vi "数据主动和反控发送2.vi"() -> ()   [LabVIEW 2016, in "数据传输系统-06.lvlib"]
uses:
  <vilib>/ptbypt/NI_PtbyPt.lvlib
panel:
  in  "N个五分钟":u32
  out "QN":string
  out "元素":cluster{"命令编码CN":string, "QN":string}[](array[cluster])
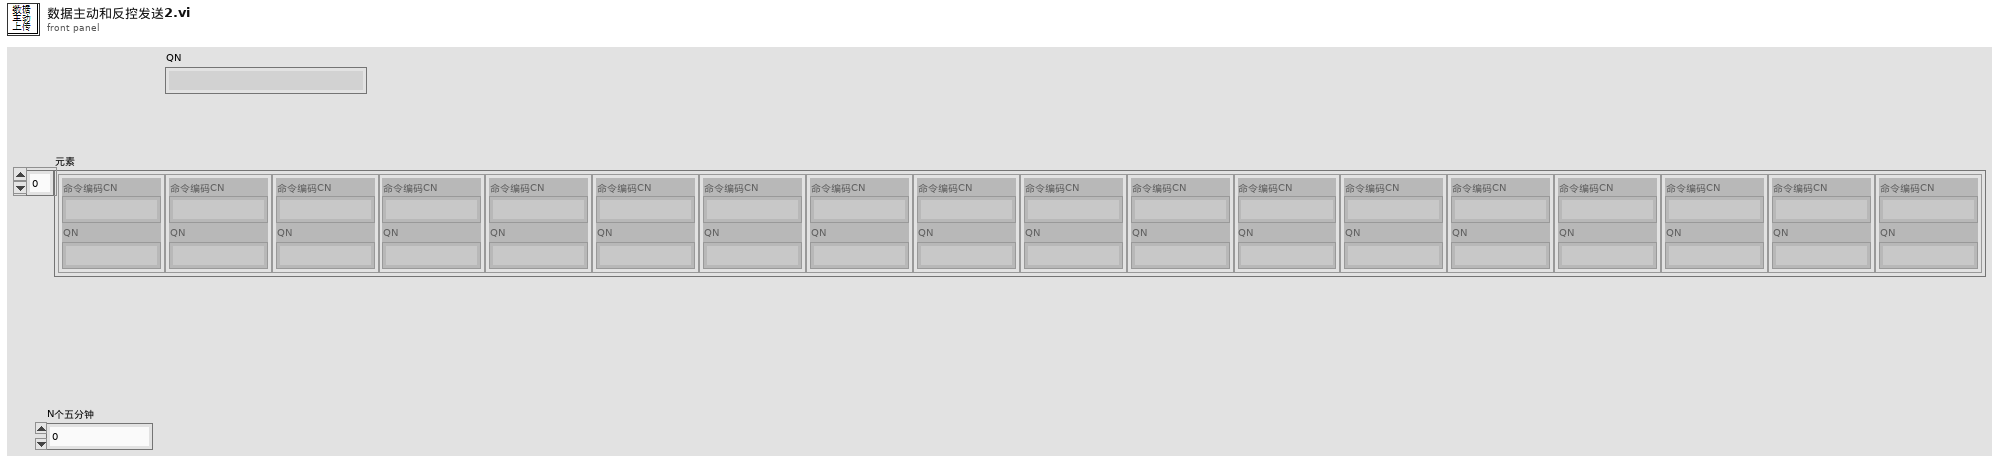
[diagram p1: front panel]
types:
  T1 = cluster{"setini":string, "sysini":string, "hechaini":string, "actualwrite":string, "actualread":string, "datasent":string, "反控命令信息队列":string, "反控与仪器交互":string}
  T2 = typedef "LVDateTimeRec.ctl" = cluster{"秒数的小数部分":dbl, "秒":i32, "分":i32, "时":i32, "日":i32, "月":i32, "年":i32, "天数（周）":i32, "天数（年）":i32, "DST":i32}
  T3 = typedef "数据传输系统-06.lvlib/应用环境.ctl" = enum16{"STD", "GB212", "婉仪平台"}
  T4 = enum16{"关闭", "星期日", "星期一", "星期二", "星期三", "星期四", "星期五", "星期六"}
  T5 = enum16{"00点", "01点", "02点", "03点", "04点", "05点", "06点", "07点", "08点", "09点", "10点", "11点", "12点", "13点", "14点", "15点", "16点", "17点", "18点", "19点", "20点", "21点", "22点", "23点"}
  T6 = cluster{"[0]":string, "[1]":string, "[2]":string, "[3]":string, "[4]":string, "[5]":string, "[6]":string, "[7]":string, "[8]":string, "[9]":string, "[10]":string, "[11]":string, "[12]":string, "[13]":string, "[14]":string, "[15]":string, "[16]":string, "[17]":string, "[18]":string, "[19]":string, "[20]":string, "[21]":string, "[22]":string, "[23]":string, "[24]":string, "[25]":string, "[26]":string, "[27]":string, "[28]":string, "[29]":string, "[30]":string, "[31]":string, "[32]":string, "[33]":string, "[34]":string, "[35]":string, "[36]":string, "[37]":string, "[38]":string, "[39]":string, "[40]":string, "[41]":string, "[42]":string, "[43]":string, "[44]":string, "[45]":string, "[46]":string, "[47]":string, "[48]":string, "[49]":string, "[50]":string, "[51]":string, "[52]":string, "[53]":string, "[54]":string, "[55]":string, "[56]":string, "[57]":string, "[58]":string, "[59]":string, "[60]":string, "[61]":string, "[62]":string, "[63]":string, "[64]":string, "[65]":string, "[66]":string, "[67]":string, "[68]":string, "[69]":string, "[70]":string, "[71]":string, "[72]":string, "[73]":string, "[74]":string, "[75]":string}
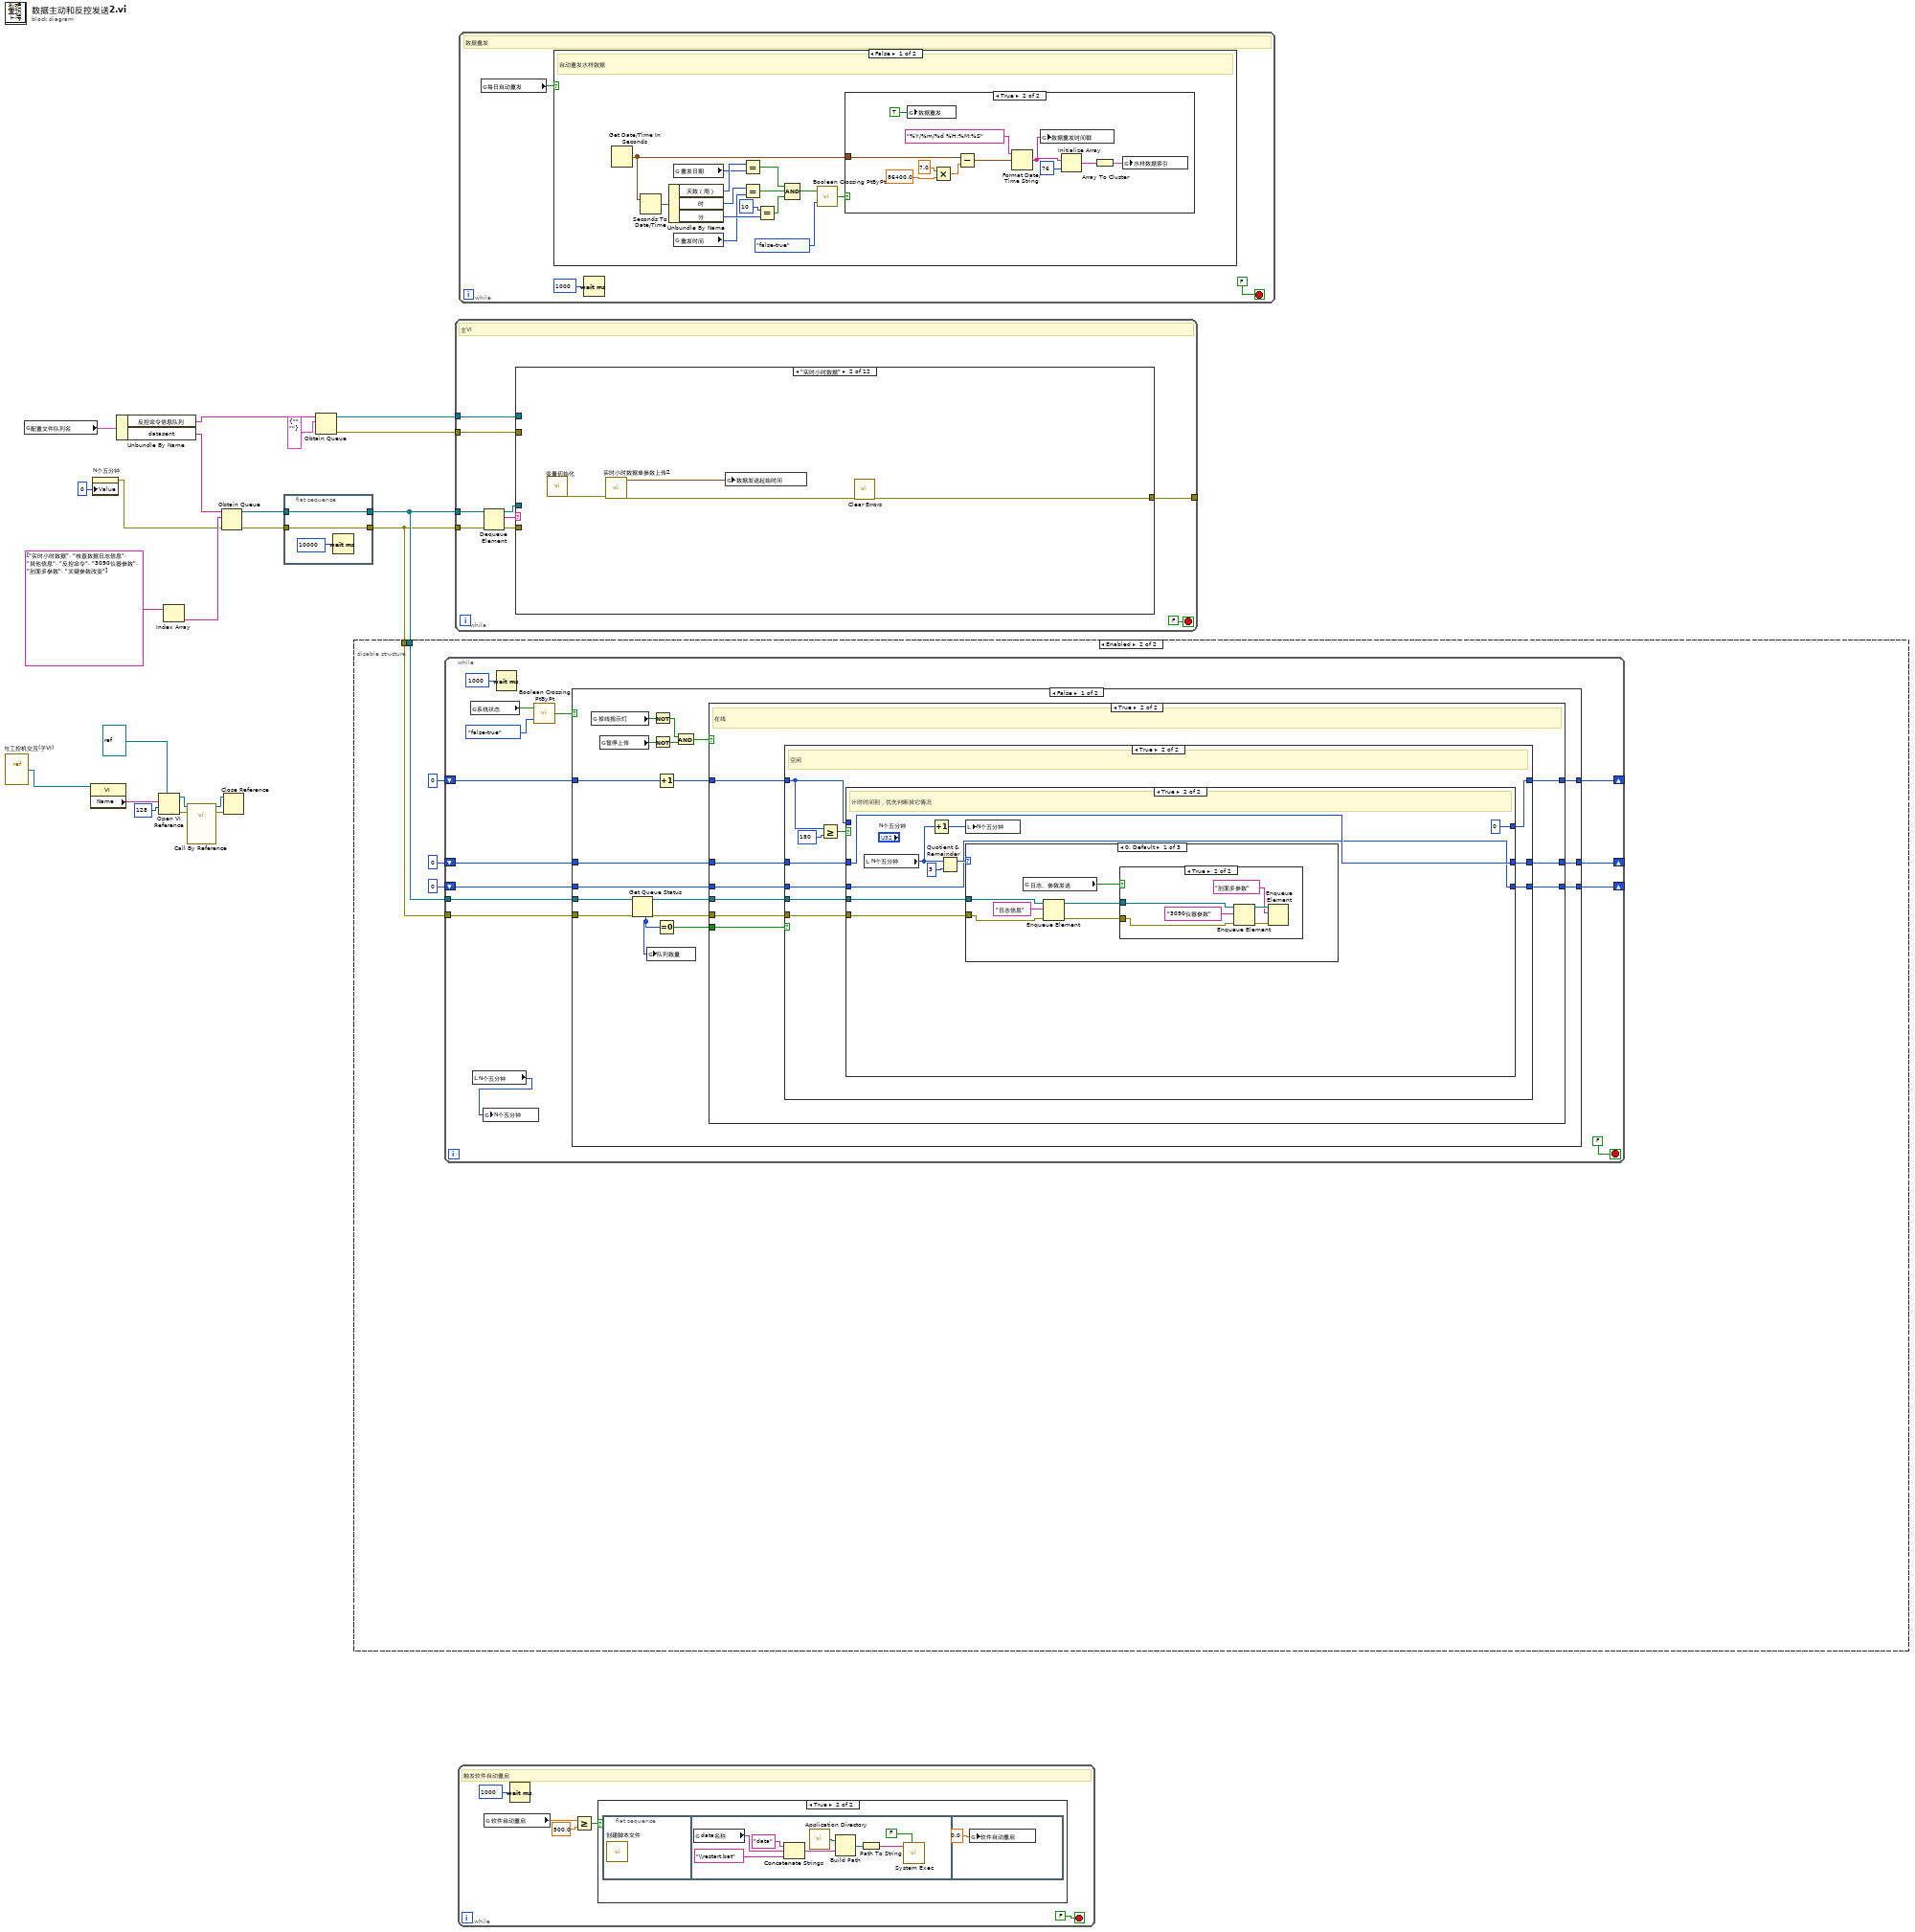
[diagram p0: block diagram]
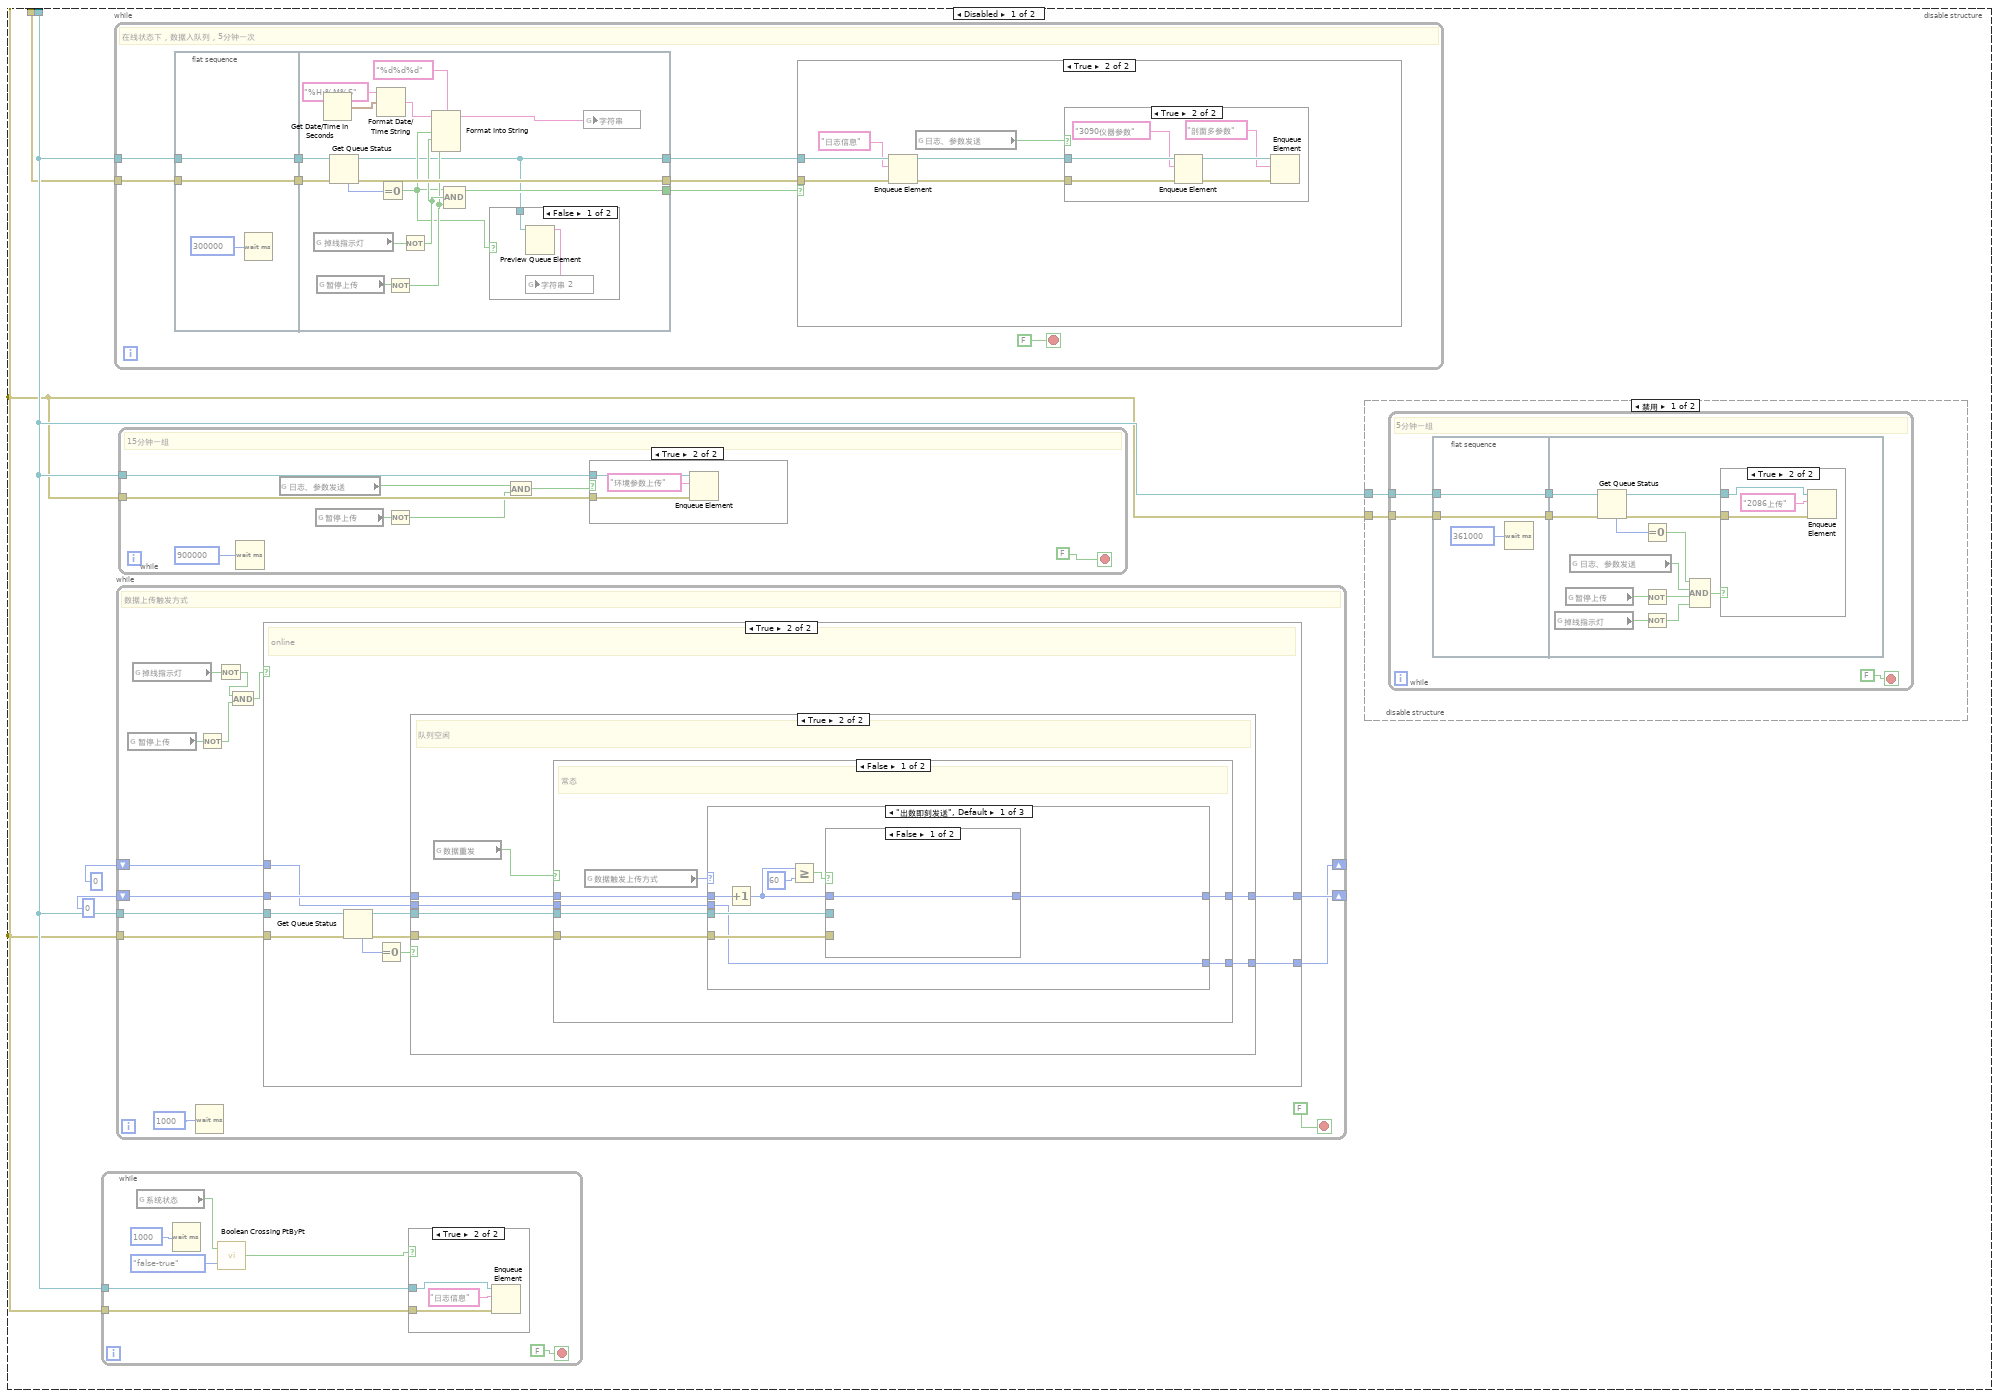
[diagram p2: hidden frame]
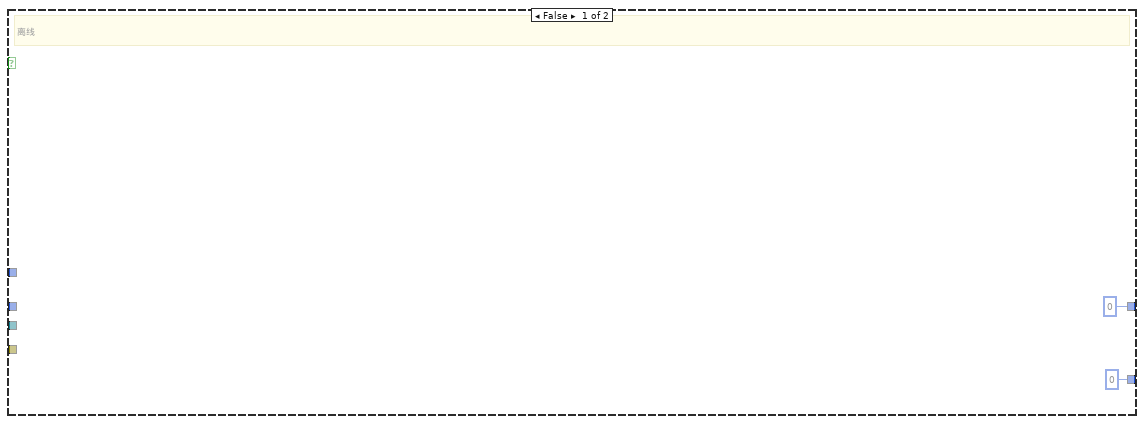
[diagram p6: hidden frame]
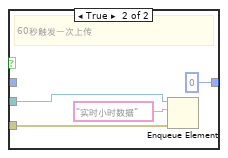
[diagram p8: hidden frame]
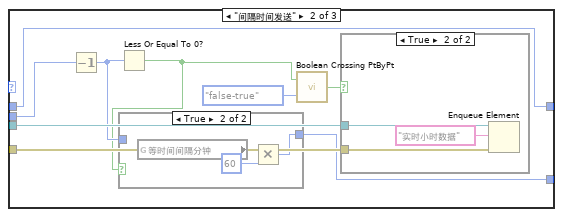
[diagram p9: hidden frame]
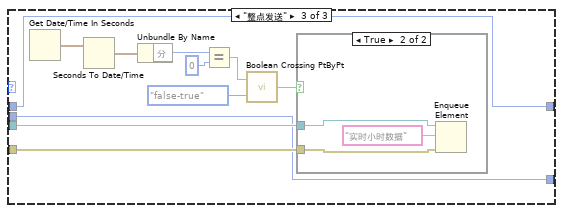
[diagram p12: hidden frame]
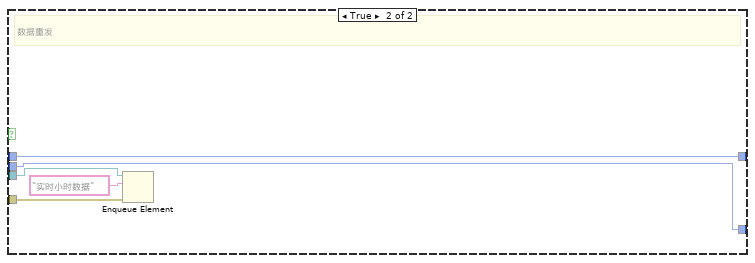
[diagram p14: hidden frame]
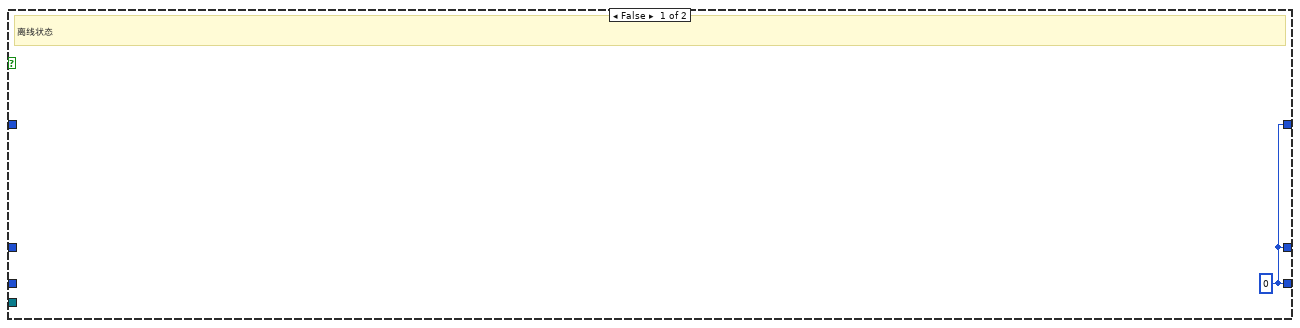
[diagram p19: hidden frame]
diagram:
  n1 = vi-ref "与工控机交互(子VI).vi"() -> (w15:refnum<vi>)
  n2 = global read "全局1.vi" "配置文件队列名"() -> (w5:T1)
  n3 = property class="VI"(reference=w15) -> ("Name"=w14:string)  [unwired: 1 in, 2 out]
  n4 = property on="N个五分钟" class="DigNum (strict)"("Value"=u32 0 ("N个五分钟")) -> (error out=w1:errorcluster)  [unwired: 2 in, 1 out]
  n5 = Unbundle By Name(w5) -> ("反控命令信息队列"=w9:string, "datasent"=w8:string)
  n6 = Open VI Reference(type specifier VI Refnum (for type only)=refnum<vi> refnum, vi path=w14, options=128 ("选项")) -> (vi reference=w12:refnum<vi>, error out=w6:errorcluster)  [unwired: 3 in]
  n7 = Index Array(array=string[] ["实时小时数据", "核查数据日志信息", "其他信息", "反控命令", "3090仪器参数", "剖面多参数", "关键参数改变"]) -> (element=w16:string)  [unwired: 1 in]
  n8 = call-by-ref "?"(reference=w12, error in=w6) -> (reference out=w10:refnum<vi>, error out=w7:errorcluster)  [unwired: 12 in]
  n9 = Obtain Queue(name (unnamed)=w8, element data type=w16, error in (no error)=w1) -> (queue out=w22:refnum<queue>, error out=w21:errorcluster)  [unwired: 2 in, 1 out]
  n10 = Close Reference(reference=w10, error in (no error)=w7) -> ()  [unwired: 1 out]
  n11 = flat-sequence {
    tunnel: w22 -> [w24]
    tunnel: [w24] -> w4
    tunnel: w21 -> [w23]
    tunnel: [w23] -> w3
    frame #0 {
      n12 = Wait (ms)(milliseconds to wait=u32 10000 ("等待时间（毫秒）")) -> ()  [unwired: 1 out]
    }
  }
  n13 = Obtain Queue(name (unnamed)=w9, element data type=cluster{"命令编码CN":string, "QN":string} {"命令编码CN"="", "QN"=""}) -> (queue out=w19:refnum<queue>, error out=w18:errorcluster)  [unwired: 3 in, 1 out]
  n14 = disable-structure shown="Enabled" {
    disable-tunnel: w4 -> [w27 w210]
    disable-tunnel: w3 -> [w26 w209]
    frame Disabled {
      n15 = while {
        tunnel: w27 -> [w57]
        tunnel: w26 -> [w56]
        stop <- FALSE stop-if-true
        n16 = global read "全局1.vi" "系统状态"() -> (w59:bool)
        n17 = Wait (ms)(milliseconds to wait=u32 1000 ("等待时间（毫秒）")) -> ()  [unwired: 1 out]
        n18 = call <vilib>:"Boolean Crossing PtByPt.vi"("direction"=enum16{"either", "false-true", "true-false"}."false-true", "input"=w59) -> ("crossing"=w55:bool)  [unwired: 1 in]
        n19 = case shown="True" w55 {
          tunnel: w57 -> [_ w62]
          tunnel: w56 -> [_ w63]
          frame False {
          }
          frame True {
            n20 = Enqueue Element(queue=w62, element="日志信息" ("元素"), error in (no error)=w63) -> ()  [unwired: 1 in, 3 out]
          }
        }
      }
      n21 = while {
        tunnel: w27 -> [w172]
        tunnel: w26 -> [w171]
        stop <- FALSE stop-if-true
        # "在线状态下，数据入队列，5分钟一次"
        n22 = flat-sequence {
          tunnel: w171 -> [w174]
          tunnel: w172 -> [w175]
          tunnel: [w175] -> w166
          tunnel: [w174] -> w165
          tunnel: [w177] -> w170
          tunnel: [w189] -> w169
          tunnel: [w187] -> w167
          tunnel: w166 -> [w191]
          tunnel: w165 -> [w190]
          frame #0 {
            n23 = Wait (ms)(milliseconds to wait=u32 300000 ("等待时间（毫秒）")) -> ()  [unwired: 1 out]
          }
          frame #1 {
            n24 = global read "全局 数据发送重叠.vi" "掉线指示灯"() -> (w188:bool)
            n25 = global read "断电保存全局.vi" "暂停上传"() -> (w186:bool)
            n26 = Get Date/Time In Seconds() -> (seconds since 1Jan1904=w184:timestamp)
            n27 = Get Queue Status(queue=w191, error in (no error)=w190) -> (queue out=w177:refnum<queue>, error out=w189:errorcluster, # elements in queue=w185:i32)  [unwired: 1 in, 5 out]
            n28 = Format Date/Time String(time format string (%c)="%H:%M%S" ("时间格式字符串(%c)"), seconds (now)=w184) -> (date/time string=w182:string)  [unwired: 1 in]
            n29 = Equal To 0?(x=w185) -> (x = 0?=w178:bool)
            n30 = Not(x=w186) -> (.not. x?=w179:bool)
            n31 = Not(x=w188) -> (.not. x?=w180:bool)
            n32 = Format Into String(format string="%d%d%d" ("格式字符串"), initial string=w182, w178, w180, w179) -> (resulting string=w176:string)  [unwired: 1 in, 1 out]
            n33 = Compound Arithmetic op=AND ("复合运算")(w178, w180, w179) -> (w187:bool)
            n34 = case shown="False" w178 {
              tunnel: w177 -> [w193 _]
              frame False {
                n35 = Preview Queue Element(queue=w193) -> (element=w192:string)  [unwired: 2 in, 3 out]
                n36 = global write "全局 水样时间.vi" "字符串 2"(w192) -> ()
              }
              frame True {
              }
            }
            n37 = global write "全局 水样时间.vi" "字符串"(w176) -> ()
          }
        }
        n38 = case shown="True" w167 {
          tunnel: w170 -> [_ w199]
          tunnel: w169 -> [_ w198]
          frame False {
          }
          frame True {
            n39 = Enqueue Element(queue=w199, element="日志信息" ("元素"), error in (no error)=w198) -> (queue out=w196:refnum<queue>, error out=w195:errorcluster)  [unwired: 1 in, 1 out]
            n40 = global read "断电保存全局.vi" "日志、参数发送"() -> (w194:bool)
            n41 = case shown="True" w194 {
              tunnel: w196 -> [_ w205]
              tunnel: w195 -> [_ w204]
              frame False {
              }
              frame True {
                n42 = Enqueue Element(queue=w205, element="3090仪器参数" ("元素"), error in (no error)=w204) -> (queue out=w202:refnum<queue>, error out=w201:errorcluster)  [unwired: 1 in, 1 out]
                n43 = Enqueue Element(queue=w202, element="剖面多参数" ("元素"), error in (no error)=w201) -> ()  [unwired: 1 in, 3 out]
              }
            }
          }
        }
      }
      n44 = while {
        tunnel: w27 -> [w72]
        tunnel: w26 -> [w71]
        shift-right: [w74] -> _
        shift-left: 0 -> [w75]
        shift-right: [w65] -> _
        shift-left: 0 -> [w66]
        stop <- FALSE stop-if-true
        # "数据上传触发方式"
        n45 = global read "断电保存全局.vi" "暂停上传"() -> (w69:bool)
        n46 = global read "全局 数据发送重叠.vi" "掉线指示灯"() -> (w76:bool)
        n47 = Wait (ms)(milliseconds to wait=u32 1000 ("等待时间（毫秒）")) -> ()  [unwired: 1 out]
        n48 = Not(x=w69) -> (.not. x?=w68:bool)
        n49 = Not(x=w76) -> (.not. x?=w70:bool)
        n50 = And(x=w70, y=w68) -> (x .and. y?=w67:bool)
        n51 = case shown="True" w67 {
          tunnel: w75 -> [_ w89]
          tunnel: [0 w88] -> w74
          tunnel: w72 -> [_ w86]
          tunnel: w71 -> [_ w85]
          tunnel: w66 -> [_ w81]
          tunnel: [0 w80] -> w65
          frame False {
            # "离线"
          }
          frame True {
            # "online"
            n52 = Get Queue Status(queue=w86, error in (no error)=w85) -> (queue out=w83:refnum<queue>, error out=w82:errorcluster, # elements in queue=w87:i32)  [unwired: 1 in, 5 out]
            n53 = Equal To 0?(x=w87) -> (x = 0?=w84:bool)
            n54 = case shown="True" w84 {
              tunnel: w83 -> [_ w98]
              tunnel: w82 -> [_ w97]
              tunnel: w89 -> [w91 w96]
              tunnel: [w91 w95] -> w88
              tunnel: w81 -> [w90 w94]
              tunnel: [w90 w93] -> w80
              frame False {
                # "队列忙碌中"
              }
              frame True {
                # "队列空闲"
                n55 = global read "断电保存全局.vi" "数据重发"() -> (w92:bool)
                n56 = case shown="False" w92 {
                  tunnel: w98 -> [w105 w152]
                  tunnel: w97 -> [w104 w151]
                  tunnel: w96 -> [w102 w150]
                  tunnel: [w101 w150] -> w95
                  tunnel: w94 -> [w100 w149]
                  tunnel: [w99 w149] -> w93
                  frame False {
                    # "常态"
                    n57 = global read "断电保存全局.vi" "数据触发上传方式"() -> (w103:enum16{"出数即刻发送", "间隔时间发送", "整点发送"})
                    n58 = case shown="\"出数即刻发送\", Default" w103 {
                      tunnel: w105 -> [w108 w126 w139]
                      tunnel: w104 -> [w107 w125 w138]
                      tunnel: w102 -> [w113 w127 w137]
                      tunnel: [w109 w127 w137] -> w101
                      tunnel: w100 -> [w106 w122 w135]
                      tunnel: [w106 w121 w135] -> w99
                      frame "出数即刻发送", Default {
                        n59 = Increment(x=w113) -> (x+1=w110:i32)
                        n60 = Greater Or Equal?(x=w110, y=60) -> (x >= y?=w111:bool)
                        n61 = case shown="False" w111 {
                          tunnel: w110 -> [w114 _]
                          tunnel: [w114 0] -> w109
                          tunnel: w108 -> [_ w116]
                          tunnel: w107 -> [_ w115]
                          frame False {
                          }
                          frame True {
                            # "60秒触发一次上传"
                            n62 = Enqueue Element(queue=w116, element="实时小时数据" ("元素"), error in (no error)=w115) -> ()  [unwired: 1 in, 3 out]
                          }
                        }
                      }
                      frame "间隔时间发送" {
                        n63 = Decrement(x=w122) -> (x-1=w120:i32)
                        n64 = Less Or Equal To 0?(x=w120) -> (x <= 0?=w119:bool)
                        n65 = case shown="True" w119 {
                          tunnel: w120 -> [w128 _]
                          tunnel: [w128 w129] -> w121
                          frame False {
                          }
                          frame True {
                            n66 = global read "断电保存全局.vi" "等时间间隔分钟"() -> (w130:i32)
                            n67 = Multiply(x=w130, y=60) -> (x*y=w129:i32)
                          }
                        }
                        n68 = call <vilib>:"Boolean Crossing PtByPt.vi"("direction"=enum16{"either", "false-true", "true-false"}."false-true", "input"=w119) -> ("crossing"=w123:bool)  [unwired: 1 in]
                        n69 = case shown="True" w123 {
                          tunnel: w126 -> [_ w133]
                          tunnel: w125 -> [_ w132]
                          frame False {
                          }
                          frame True {
                            n70 = Enqueue Element(queue=w133, element="实时小时数据" ("元素"), error in (no error)=w132) -> ()  [unwired: 1 in, 3 out]
                          }
                        }
                      }
                      frame "整点发送" {
                        n71 = Get Date/Time In Seconds() -> (seconds since 1Jan1904=w144:timestamp)
                        n72 = Seconds To Date/Time(time stamp (now)=w144) -> (date time rec=w145:T2)  [unwired: 1 in]
                        n73 = Unbundle By Name(w145) -> ("分"=w143:i32)
                        n74 = Equal?(x=w143, y=0) -> (x = y?=w141:bool)
                        n75 = call <vilib>:"Boolean Crossing PtByPt.vi"("direction"=enum16{"either", "false-true", "true-false"}."false-true", "input"=w141) -> ("crossing"=w136:bool)  [unwired: 1 in]
                        n76 = case shown="True" w136 {
                          tunnel: w139 -> [_ w147]
                          tunnel: w138 -> [_ w146]
                          frame False {
                          }
                          frame True {
                            n77 = Enqueue Element(queue=w147, element="实时小时数据" ("元素"), error in (no error)=w146) -> ()  [unwired: 1 in, 3 out]
                          }
                        }
                      }
                    }
                  }
                  frame True {
                    # "数据重发"
                    n78 = Enqueue Element(queue=w152, element="实时小时数据" ("元素"), error in (no error)=w151) -> ()  [unwired: 1 in, 3 out]
                  }
                }
              }
            }
          }
        }
      }
      n79 = while {
        tunnel: w27 -> [w159]
        tunnel: w26 -> [w158]
        stop <- FALSE stop-if-true
        # "15分钟一组"
        n80 = Wait (ms)(milliseconds to wait=u32 900000 ("等待时间（毫秒）")) -> ()  [unwired: 1 out]
        n81 = global read "断电保存全局.vi" "日志、参数发送"() -> (w156:bool)
        n82 = global read "断电保存全局.vi" "暂停上传"() -> (w157:bool)
        n83 = Not(x=w157) -> (.not. x?=w155:bool)
        n84 = And(x=w156, y=w155) -> (x .and. y?=w154:bool)
        n85 = case shown="True" w154 {
          tunnel: w159 -> [_ w163]
          tunnel: w158 -> [_ w162]
          frame False {
          }
          frame True {
            n86 = Enqueue Element(queue=w163, element="环境参数上传" ("元素"), error in (no error)=w162) -> ()  [unwired: 1 in, 3 out]
          }
        }
      }
      n87 = disable-structure shown="禁用" {
        disable-tunnel: w27 -> [w31 _]
        disable-tunnel: w26 -> [w30 _]
        frame Disabled {
          n88 = while {
            tunnel: w31 -> [w35]
            tunnel: w30 -> [w34]
            stop <- FALSE stop-if-true
            # "5分钟一组"
            n89 = flat-sequence {
              tunnel: w34 -> [w38]
              tunnel: w35 -> [w39]
              tunnel: [w39] -> w33
              tunnel: [w38] -> w32
              tunnel: w33 -> [w46]
              tunnel: w32 -> [w45]
              frame #0 {
                n90 = Wait (ms)(milliseconds to wait=u32 361000 ("等待时间（毫秒）")) -> ()  [unwired: 1 out]
              }
              frame #1 {
                n91 = global read "全局 数据发送重叠.vi" "掉线指示灯"() -> (w43:bool)
                n92 = global read "断电保存全局.vi" "暂停上传"() -> (w51:bool)
                n93 = global read "断电保存全局.vi" "日志、参数发送"() -> (w50:bool)
                n94 = Get Queue Status(queue=w46, error in (no error)=w45) -> (queue out=w44:refnum<queue>, error out=w40:errorcluster, # elements in queue=w47:i32)  [unwired: 1 in, 5 out]
                n95 = Equal To 0?(x=w47) -> (x = 0?=w41:bool)
                n96 = Not(x=w51) -> (.not. x?=w49:bool)
                n97 = Not(x=w43) -> (.not. x?=w42:bool)
                n98 = Compound Arithmetic op=AND ("复合运算")(w41, w50, w49, w42) -> (w48:bool)
                n99 = case shown="True" w48 {
                  tunnel: w44 -> [_ w53]
                  tunnel: w40 -> [_ w52]
                  frame False {
                  }
                  frame True {
                    n100 = Enqueue Element(queue=w53, element="2086上传" ("元素"), error in (no error)=w52) -> ()  [unwired: 1 in, 3 out]
                  }
                }
              }
            }
          }
        }
        frame Enabled {
        }
      }
    }
    frame Enabled {
      n101 = while {
        tunnel: w210 -> [w219]
        tunnel: w209 -> [w218]
        shift-right: [w217] -> _
        shift-left: 0 -> [w211]
        shift-right: [w216] -> _
        shift-left: 0 -> [w212]
        shift-right: [w215] -> _
        shift-left: 0 -> [w213]
        stop <- FALSE stop-if-true
        n102 = global read "全局1.vi" "系统状态"() -> (w222:bool)
        n103 = local read "N个五分钟"() -> (w214:u32)
        n104 = global write "全局 水样时间.vi" "N个五分钟"(w214) -> ()
        n105 = Wait (ms)(milliseconds to wait=u32 1000 ("等待时间（毫秒）")) -> ()  [unwired: 1 out]
        n106 = call <vilib>:"Boolean Crossing PtByPt.vi"("direction"=enum16{"either", "false-true", "true-false"}."false-true", "input"=w222) -> ("crossing"=w220:bool)  [unwired: 1 in]
        n107 = case shown="False" w220 {
          tunnel: w219 -> [w230 w360]
          tunnel: w218 -> [w229 w361]
          tunnel: [w237 w359] -> w217
          tunnel: [w236 w358] -> w216
          tunnel: w211 -> [w235 w359]
          tunnel: w212 -> [w234 w358]
          tunnel: w213 -> [w233 w357]
          tunnel: [w231 w357] -> w215
          frame False {
            n108 = global read "全局 数据发送重叠.vi" "掉线指示灯"() -> (w242:bool)
            n109 = global read "断电保存全局.vi" "暂停上传"() -> (w240:bool)
            n110 = Get Queue Status(queue=w230, error in (no error)=w229) -> (queue out=w228:refnum<queue>, error out=w227:errorcluster, # elements in queue=w225:i32)  [unwired: 1 in, 5 out]
            n111 = global write "全局 水样时间.vi" "队列数量"(w225) -> ()
            n112 = Not(x=w242) -> (.not. x?=w241:bool)
            n113 = Not(x=w240) -> (.not. x?=w239:bool)
            n114 = Increment(x=w233) -> (x+1=w232:i32)
            n115 = Equal To 0?(x=w225) -> (x = 0?=w226:bool)
            n116 = And(x=w241, y=w239) -> (x .and. y?=w238:bool)
            n117 = case shown="True" w238 {
              tunnel: [w243 w251] -> w237
              tunnel: [w243 w249] -> w236
              tunnel: w228 -> [_ w246]
              tunnel: w235 -> [_ w252]
              tunnel: w234 -> [_ w250]
              tunnel: w232 -> [_ w248]
              tunnel: [w243 w247] -> w231
              tunnel: w227 -> [_ w245]
              tunnel: w226 -> [_ w244]
              frame False {
                w243 = 0
                # "离线状态"
              }
              frame True {
                # "在线"
                n118 = case shown="True" w244 {
                  tunnel: w252 -> [w255 w261]
                  tunnel: [w255 w260] -> w251
                  tunnel: w250 -> [w254 w263]
                  tunnel: [w254 w262] -> w249
                  tunnel: w246 -> [_ w265]
                  tunnel: w245 -> [_ w264]
                  tunnel: w248 -> [w253 w256]
                  tunnel: [w253 w257] -> w247
                  frame False {
                    # "忙碌"
                  }
                  frame True {
                    # "空闲"
                    n119 = Greater Or Equal?(x=w256, y=180) -> (x >= y?=w258:bool)
                    n120 = case shown="True" w258 {
                      tunnel: w265 -> [w272 w331]
                      tunnel: w264 -> [w271 w330]
                      tunnel: w263 -> [w270 w337]
                      tunnel: [w269 w337] -> w262
                      tunnel: w261 -> [w268 w329]
                      tunnel: [w267 w329] -> w260
                      tunnel: [w266 0] -> w257
                      tunnel: w256 -> [w266 _]
                      frame False {
                        # "五分钟计时未到"
                        n121 = global read "断电保存全局.vi" "数据重发"() -> (w273:bool)
                        n122 = case shown="False" w273 {
                          tunnel: w272 -> [w278 w328]
                          tunnel: w271 -> [w277 w327]
                          tunnel: w270 -> [w279 w324]
                          tunnel: [w276 w324] -> w269
                          tunnel: w268 -> [w275 w325]
                          tunnel: [w274 w325] -> w267
                          frame False {
                            n123 = global read "断电保存全局.vi" "数据触发上传方式"() -> (w280:enum16{"出数即刻发送", "间隔时间发送", "整点发送"})
                            n124 = case shown="\"出数即刻发送\", Default" w280 {
                              tunnel: w279 -> [w288 w294 w310]
                              tunnel: w278 -> [w285 w297 w313]
                              tunnel: w277 -> [w284 w296 w312]
                              tunnel: [w283 w294 w310] -> w276
                              tunnel: w275 -> [w282 w301 w311]
                              tunnel: [w282 w295 w311] -> w274
                              frame "出数即刻发送", Default {
                                n125 = Increment(x=w288) -> (x+1=w281:i32)
                                n126 = Greater Or Equal?(x=w281, y=60) -> (x >= y?=w286:bool)
                                n127 = case shown="True" w286 {
                                tunnel: w285 -> [_ w293]
                                tunnel: w284 -> [_ w292]
                                tunnel: [w289 0] -> w283
                                tunnel: w281 -> [w289 _]
                                frame False {
                                }
                                frame True {
                                n128 = Enqueue Element(queue=w293, element="实时小时数据", error in (no error)=w292) -> ()  [unwired: 1 in, 3 out]
                                }
                                }
                              }
                              frame "间隔时间发送" {
                                n129 = Decrement(x=w301) -> (x-1=w300:i32)
                                n130 = Less Or Equal To 0?(x=w300) -> (x <= 0?=w299:bool)
                                n131 = case shown="True" w299 {
                                tunnel: w300 -> [w306 _]
                                tunnel: [w306 w307] -> w295
                                frame False {
                                }
                                frame True {
                                n132 = global read "断电保存全局.vi" "等时间间隔分钟"() -> (w308:i32)
                                n133 = Multiply(x=w308, y=60) -> (x*y=w307:i32)
                                }
                                }
                                n134 = call <vilib>:"Boolean Crossing PtByPt.vi"("direction"=enum16{"either", "false-true", "true-false"}."false-true", "input"=w299) -> ("crossing"=w298:bool)  [unwired: 1 in]
                                n135 = case shown="True" w298 {
                                tunnel: w297 -> [_ w304]
                                tunnel: w296 -> [_ w303]
                                frame False {
                                }
                                frame True {
                                n136 = Enqueue Element(queue=w304, element="实时小时数据" ("元素"), error in (no error)=w303) -> ()  [unwired: 1 in, 3 out]
                                }
                                }
                              }
                              frame "整点发送" {
                                n137 = Get Date/Time In Seconds() -> (seconds since 1Jan1904=w316:timestamp)
                                n138 = Seconds To Date/Time(time stamp (now)=w316) -> (date time rec=w315:T2)  [unwired: 1 in]
                                n139 = Unbundle By Name(w315) -> ("分"=w317:i32)
                                n140 = Equal?(x=w317, y=0) -> (x = y?=w319:bool)
                                n141 = call <vilib>:"Boolean Crossing PtByPt.vi"("direction"=enum16{"either", "false-true", "true-false"}."false-true", "input"=w319) -> ("crossing"=w314:bool)  [unwired: 1 in]
                                n142 = case shown="True" w314 {
                                tunnel: w313 -> [_ w322]
                                tunnel: w312 -> [_ w321]
                                frame False {
                                }
                                frame True {
                                n143 = Enqueue Element(queue=w322, element="实时小时数据" ("元素"), error in (no error)=w321) -> ()  [unwired: 1 in, 3 out]
                                }
                                }
                              }
                            }
                          }
                          frame True {
                            n144 = Enqueue Element(queue=w328, element="实时小时数据" ("元素"), error in (no error)=w327) -> ()  [unwired: 1 in, 3 out]
                          }
                        }
                      }
                      frame True {
                        # "计时时间到，优先判断其它情况"
                        n145 = local read "N个五分钟"() -> (w332:u32)
                        n146 = Increment(x=w332) -> (x+1=w333:u32)
                        n147 = Quotient & Remainder(x=w332, y=u32 3) -> (x-y*floor(x/y)=w334:u32)  [unwired: 1 out]
                        n148 = local write "N个五分钟"(w333) -> ()
                        n149 = case shown="0, Default" w334 {
                          tunnel: w331 -> [w339 w352 w354]
                          tunnel: w330 -> [w338 w351 w355]
                          frame 0, Default {
                            n150 = global read "断电保存全局.vi" "日志、参数发送"() -> (w343:bool)
                            n151 = Enqueue Element(queue=w339, element="日志信息" ("元素"), error in (no error)=w338) -> (queue out=w341:refnum<queue>, error out=w342:errorcluster)  [unwired: 1 in, 1 out]
                            n152 = case shown="True" w343 {
                              tunnel: w341 -> [_ w349]
                              tunnel: w342 -> [_ w348]
                              frame False {
                              }
                              frame True {
                                n153 = Enqueue Element(queue=w349, element="3090仪器参数" ("元素"), error in (no error)=w348) -> (queue out=w346:refnum<queue>, error out=w345:errorcluster)  [unwired: 1 in, 1 out]
                                n154 = Enqueue Element(queue=w346, element="剖面多参数" ("元素"), error in (no error)=w345) -> ()  [unwired: 1 in, 3 out]
                              }
                            }
                          }
                          frame 1 {
                            n155 = Enqueue Element(queue=w352, element="2086上传" ("元素"), error in (no error)=w351) -> ()  [unwired: 1 in, 3 out]
                            n156 = global write "全局1.vi" "2086上传"(TRUE ("2086上传")) -> ()
                          }
                          frame 2 {
                            n157 = Enqueue Element(queue=w354, element="环境参数上传" ("元素"), error in (no error)=w355) -> ()  [unwired: 1 in, 3 out]
                          }
                        }
                      }
                    }
                  }
                }
              }
            }
          }
          frame True {
            n158 = Enqueue Element(queue=w360, element="日志信息" ("元素"), error in (no error)=w361) -> ()  [unwired: 1 in, 3 out]
          }
        }
      }
    }
  }
  n159 = while {
    tunnel: w4 -> [w365]
    tunnel: w3 -> [w364]
    tunnel: w19 -> [w367]
    tunnel: w18 -> [w366]
    tunnel: [w363] -> _
    stop <- FALSE stop-if-true
    # "主VI"
    n160 = Dequeue Element(queue=w365, error in (no error)=w364) -> (queue out=w369:refnum<queue>, element=w370:string, error out=w368:errorcluster)  [unwired: 1 in, 1 out]
    n161 = case shown="\"实时小时数据\"" w370 {
      tunnel: w369 -> [_ _ w378 _ _ _ _ w400 _ _ _ _]
      tunnel: w368 -> [_ _ _ _ _ _ _ w399 _ _ _ _]
      tunnel: w367 -> [_ _ _ _ _ _ _ w407 _ _ _ _]
      tunnel: w366 -> [_ _ _ _ _ _ _ w406 _ _ _ _]
      tunnel: [_ w372 w377 w384 w390 w395 _ _ w420 w426 w433 _] -> w363
      frame Default {
      }
      frame "实时小时数据" {
        n162 = call "变量初始化.vi"() -> ("错误输出"=w373:errorcluster)  [unwired: 11 in]
        n163 = call "实时小时数据单参数上传2.vi"("错误输入（无错误）"=w373) -> ("数据发送起始时间"=w375:timestamp, "error out"=w374:errorcluster)  [unwired: 13 in]
        n164 = global write "全局1.vi" "数据发送起始时间"(w375) -> ()
        n165 = call <vilib>:"Clear Errors.vi"("error in (no error)"=w374) -> ("error out"=w372:errorcluster)  [unwired: 5 in, 1 out]
      }
      frame "日志信息" {
        n166 = call "日志信息出发送队列 (子VI).vi"("queue out"=w378) -> ("错误输出"=w376:errorcluster)  [unwired: 10 in]
        n167 = call <vilib>:"Clear Errors.vi"("error in (no error)"=w376) -> ("error out"=w377:errorcluster)  [unwired: 5 in, 1 out]
      }
      frame "关键参数改变" {
        n168 = global read "断电保存全局.vi" "仪器参数发送"() -> (w382:bool)
        n169 = global read "断电保存全局.vi" "应用环境"() -> (w383:T3)
        n170 = Equal?(x=w383, y=应用环境."STD" ("应用环境")) -> (x = y?=w381:bool)
        n171 = And(x=w382, y=w381) -> (x .and. y?=w380:bool)
        n172 = case shown="True" w380 {
          tunnel: [_ w385] -> w384
          frame False {
          }
          frame True {
            n173 = call "仪器参数改变发送 (子VI).vi"() -> ("错误输出"=w386:errorcluster)  [unwired: 11 in]
            n174 = call "采配水仪器参数改变发送 (子VI).vi"("错误输入"=w386) -> ("错误输出"=w385:errorcluster)  [unwired: 10 in]
          }
        }
      }
      frame "校准信息改变" {
        n175 = global read "断电保存全局.vi" "应用环境"() -> (w389:T3)
        n176 = Equal?(x=w389, y=应用环境."STD" ("应用环境")) -> (x = y?=w388:bool)
        n177 = case shown="True" w388 {
          tunnel: [_ w391] -> w390
          frame False {
          }
          frame True {
            n178 = call "校准信息改变发送 (子VI).vi"() -> ("错误输出"=w391:errorcluster)  [unwired: 11 in]
          }
        }
      }
      frame "3201告警信息改变" {
        n179 = global read "断电保存全局.vi" "应用环境"() -> (w394:T3)
        n180 = Equal?(x=w394, y=应用环境."婉仪平台") -> (x = y?=w393:bool)
        n181 = case shown="True" w393 {
          tunnel: [_ w396] -> w395
          frame False {
          }
          frame True {
            n182 = call "3201告警信息改变发送 (子VI).vi"() -> ("错误输出"=w396:errorcluster)  [unwired: 11 in]
          }
        }
      }
      frame "其他信息" {
      }
      frame "反控命令" {
        n183 = Get Queue Status(queue=w407, return elements? (F)=TRUE ("返回元素？(F)"), error in (no error)=w406) -> (elements=→"元素":cluster{"命令编码CN":string, "QN":string}[])  [unwired: 7 out]
        n184 = Dequeue Element(queue=w407, error in (no error)=w406) -> (element=w403:cluster{"命令编码CN":string, "QN":string})  [unwired: 1 in, 3 out]
        n185 = Unbundle By Name(w403) -> ("命令编码CN"=w397:string, "QN"=w398:string)
        "QN" <- w398
        n186 = global read "全局1.vi" "数据"() -> (w405:string)
        n187 = call "读取反控数据解析(子VI).vi"("数据"=w405, "命令编码CN"=w397) -> ("反控命令错误？"=w404:bool)  [unwired: 8 in, 1 out]
        n188 = case shown="False" w404 {
          tunnel: w398 -> [w412 _]
          tunnel: w400 -> [w410 _]
          tunnel: w399 -> [w409 _]
          tunnel: w397 -> [w408 _]
          frame False {
            # "反控命令正确"
            n189 = call "反控数据上传(子VI).vi"("QN"=w412) -> ("error out"=w411:errorcluster)  [unwired: 10 in]
            n190 = case shown="No Error" w411 {
              tunnel: w410 -> [w415 _]
              tunnel: w409 -> [w414 _]
              tunnel: w408 -> [w413 _]
              frame No Error {
                n191 = case shown="\"2084\", \"3056\"" w413 {
                  tunnel: w415 -> [_ w418]
                  tunnel: w414 -> [_ w417]
                  frame "假", Default {
                  }
                  frame "2084", "3056" {
                    n192 = Enqueue Element(queue=w418, element="日志信息" ("元素"), error in (no error)=w417) -> ()  [unwired: 1 in, 3 out]
                  }
                }
              }
              frame Error {
              }
            }
          }
          frame True {
            # "反控命令错误"
          }
        }
      }
      frame "3090仪器参数" {
        n193 = global read "断电保存全局.vi" "应用环境"() -> (w419:T3)
        n194 = case shown="\"STD\"" w419 {
          tunnel: [w421 _] -> w420
          frame "STD" {
            n195 = call "3090仪器参数上传.vi"() -> ("error out"=w422:errorcluster)  [unwired: 15 in]
            n196 = call "变量初始化.vi"("错误输入（无错误）"=w422) -> ("错误输出"=w421:errorcluster)  [unwired: 10 in]
          }
          frame "GB212", Default {
          }
        }
      }
      frame "剖面多参数" {
        n197 = global read "断电保存全局.vi" "应用环境"() -> (w425:T3)
        n198 = call "剖面多参数上传.vi"() -> ("error out"=w424:errorcluster)  [unwired: 15 in]
        n199 = call <vilib>:"Clear Errors.vi"("error in (no error)"=w424) -> ("error out"=w423:errorcluster)  [unwired: 5 in, 1 out]
        n200 = case shown="\"STD\"" w425 {
          tunnel: [w428 w429 w432] -> w426
          tunnel: w423 -> [w427 w429 w431]
          frame "STD" {
            n201 = call "新剖面数据上传.vi"("错误输入（无错误）"=w427) -> ("error out"=w428:errorcluster)  [unwired: 14 in]
          }
          frame "GB212", Default {
            n202 = global write "断电保存全局.vi" "剖面数据重发"(FALSE ("剖面数据重发")) -> ()
          }
          frame "婉仪平台" {
            n203 = call "新剖面数据上传.vi"("错误输入（无错误）"=w431) -> ("error out"=w432:errorcluster)  [unwired: 14 in]
          }
        }
      }
      frame "环境参数上传" {
        n204 = call "环境参数上传.vi"() -> ("error out"=w433:errorcluster)  [unwired: 15 in]
      }
      frame "2086上传" {
        n205 = flat-sequence {
          frame #0 {
            n206 = call "2086发送2.vi"() -> ()  [unwired: 12 in]
          }
          frame #1 {
            n207 = call "2086组合发送波浪仪.vi"() -> ()  [unwired: 12 in]
          }
          frame #2 {
            n208 = global write "全局1.vi" "2086上传"(FALSE ("2086上传")) -> ()
          }
        }
      }
    }
  }
  n209 = while {
    stop <- FALSE stop-if-true
    # "触发软件自动重启"
    n210 = global read "全局1.vi" "软件自动重启"() -> (w437:dbl)
    n211 = Wait (ms)(milliseconds to wait=u32 1000 ("等待时间（毫秒）")) -> ()  [unwired: 1 out]
    n212 = Greater Or Equal?(x=w437, y=500.0) -> (x >= y?=w435:bool)
    n213 = case shown="True" w435 {
      frame False {
      }
      frame True {
        n214 = flat-sequence {
          frame #0 {
            n215 = call "创建脚本文件.vi"() -> ()  [unwired: 11 in, 1 out]
          }
          frame #1 {
            n216 = global read "断电保存全局.vi" "data名称"() -> (w442:string)
            n217 = Concatenate Strings("data" ("名称或相对路径"), w442, "\\restart.bat" ("字符串")) -> (w440:string)
            n218 = call <vilib>:"Application Directory.vi"() -> ("Application Directory"=w446:path)
            n219 = Build Path(base path=w446, name or relative path=w440) -> (appended path=w447:path)
            n220 = Path To String(path=w447) -> (string=w444:string)
            n221 = call <vilib>:"System Exec.vi"("wait until completion? (T)"=FALSE, "command line"=w444) -> ()  [unwired: 6 in, 4 out]
          }
          frame #2 {
            n222 = global write "全局1.vi" "软件自动重启"(0.0 ("软件自动重启")) -> ()
          }
        }
      }
    }
  }
  n223 = while {
    stop <- FALSE stop-if-true
    # "数据重发"
    n224 = global read "断电保存全局.vi" "每日自动重发"() -> (w450:bool)
    n225 = case shown="False" w450 {
      frame False {
        # "自动重发水样数据"
        n226 = Get Date/Time In Seconds() -> (seconds since 1Jan1904=w453:timestamp)
        n227 = Seconds To Date/Time(time stamp (now)=w453) -> (date time rec=w460:T2)  [unwired: 1 in]
        n228 = Unbundle By Name(w460) -> ("天数（周）"=w465:i32, "时"=w456:i32, "分"=w464:i32)
        n229 = global read "断电保存全局.vi" "重发日期"() -> (w455:T4)
        n230 = global read "断电保存全局.vi" "重发时间"() -> (w454:T5)
        n231 = Equal?(x=w465, y=w455) -> (x = y?=w463:bool)
        n232 = Equal?(x=w456, y=w454) -> (x = y?=w462:bool)
        n233 = Equal?(x=10, y=w464) -> (x = y?=w461:bool)
        n234 = Compound Arithmetic op=AND ("复合运算")(w463, w462, w461) -> (w459:bool)
        n235 = call <vilib>:"Boolean Crossing PtByPt.vi"("direction"=enum16{"either", "false-true", "true-false"}."false-true", "input"=w459) -> ("crossing"=w458:bool)  [unwired: 1 in]
        n236 = case shown="True" w458 {
          tunnel: w453 -> [_ w467]
          frame False {
          }
          frame True {
            n237 = global write "断电保存全局.vi" "数据重发"(TRUE ("数据重发")) -> ()
            n238 = Multiply(x=7.0, y=86400.0) -> (x*y=w469:dbl)
            n239 = Subtract(x=w467, y=w469) -> (x-y=w466:timestamp)
            n240 = Format Date/Time String(time format string (%c)="%Y/%m/%d %H:%M:%S" ("时间格式字符串(%c)"), seconds (now)=w466) -> (date/time string=w471:string)  [unwired: 1 in]
            n241 = global write "断电保存全局.vi" "数据重发时间戳"(w471) -> ()
            n242 = Initialize Array(w471, 76 ("维数大小")) -> (w473:string[])
            n243 = Array To Cluster(array=w473) -> (cluster=w472:T6)
            n244 = global write "全局 水样时间.vi" "水样数据索引"(w472) -> ()
          }
        }
      }
      frame True {
        n245 = Get Date/Time In Seconds() -> (seconds since 1Jan1904=w477:timestamp)
        n246 = Seconds To Date/Time(time stamp (now)=w477) -> (date time rec=w484:T2)  [unwired: 1 in]
        n247 = global read "断电保存全局.vi" "重发时间"() -> (w479:T5)
        n248 = Unbundle By Name(w484) -> ("时"=w480:i32, "分"=w487:i32)
        n249 = Equal?(x=w480, y=w479) -> (x = y?=w486:bool)
        n250 = Equal?(x=10, y=w487) -> (x = y?=w485:bool)
        n251 = Compound Arithmetic op=AND ("复合运算")(w486, w485) -> (w483:bool)
        n252 = call <vilib>:"Boolean Crossing PtByPt.vi"("direction"=enum16{"either", "false-true", "true-false"}."false-true", "input"=w483) -> ("crossing"=w482:bool)  [unwired: 1 in]
        n253 = case shown="True" w482 {
          tunnel: w477 -> [_ w489]
          frame False {
          }
          frame True {
            n254 = global write "断电保存全局.vi" "数据重发"(TRUE ("数据重发")) -> ()
            n255 = Subtract(x=w489, y=86400.0) -> (x-y=w488:timestamp)
            n256 = Format Date/Time String(time format string (%c)="%Y/%m/%d %H:%M:%S" ("时间格式字符串(%c)"), seconds (now)=w488) -> (date/time string=w491:string)  [unwired: 1 in]
            n257 = global write "断电保存全局.vi" "数据重发时间戳"(w491) -> ()
            n258 = Initialize Array(w491, 76 ("维数大小")) -> (w493:string[])
            n259 = Array To Cluster(array=w493) -> (cluster=w492:T6)
            n260 = global write "全局 水样时间.vi" "水样数据索引"(w492) -> ()
          }
        }
      }
    }
    n261 = Wait (ms)(milliseconds to wait=u32 1000 ("等待时间（毫秒）")) -> ()  [unwired: 1 out]
  }
